vi "Obtain cycle time.vi"(8 "error in (no error)":errorcluster, 11 "Functional Imging UI Refs":T1) -> (0 "error out":errorcluster, 1 "Funct Acq Cycle time (sec)":dbl, 2 "Funct Acq cycle length (us)":dbl, 3 "Single funct.acq cycle time-stamps (us) [MovCor only]":dbl[](array[numeric]), 5 "MovCor enabled (value from header file)":bool)   [LabVIEW 2017]
uses:
  Typedefs/Functional Imging UI Refs.ctl
  xcontrol/XGrapher.xctl
  Typedefs/ROI selector array-ROI vis.ctl
  xcontrol/Interface VIs/Interface typedefs/Interface-ROI selection cluster.ctl
  Typedefs/ROI ID Enum.ctl
  Typedefs/Groups array referecne.ctl
  Typedefs/ROI visibility mode.ctl
panel:
  # "[Groups] is a Typedef"
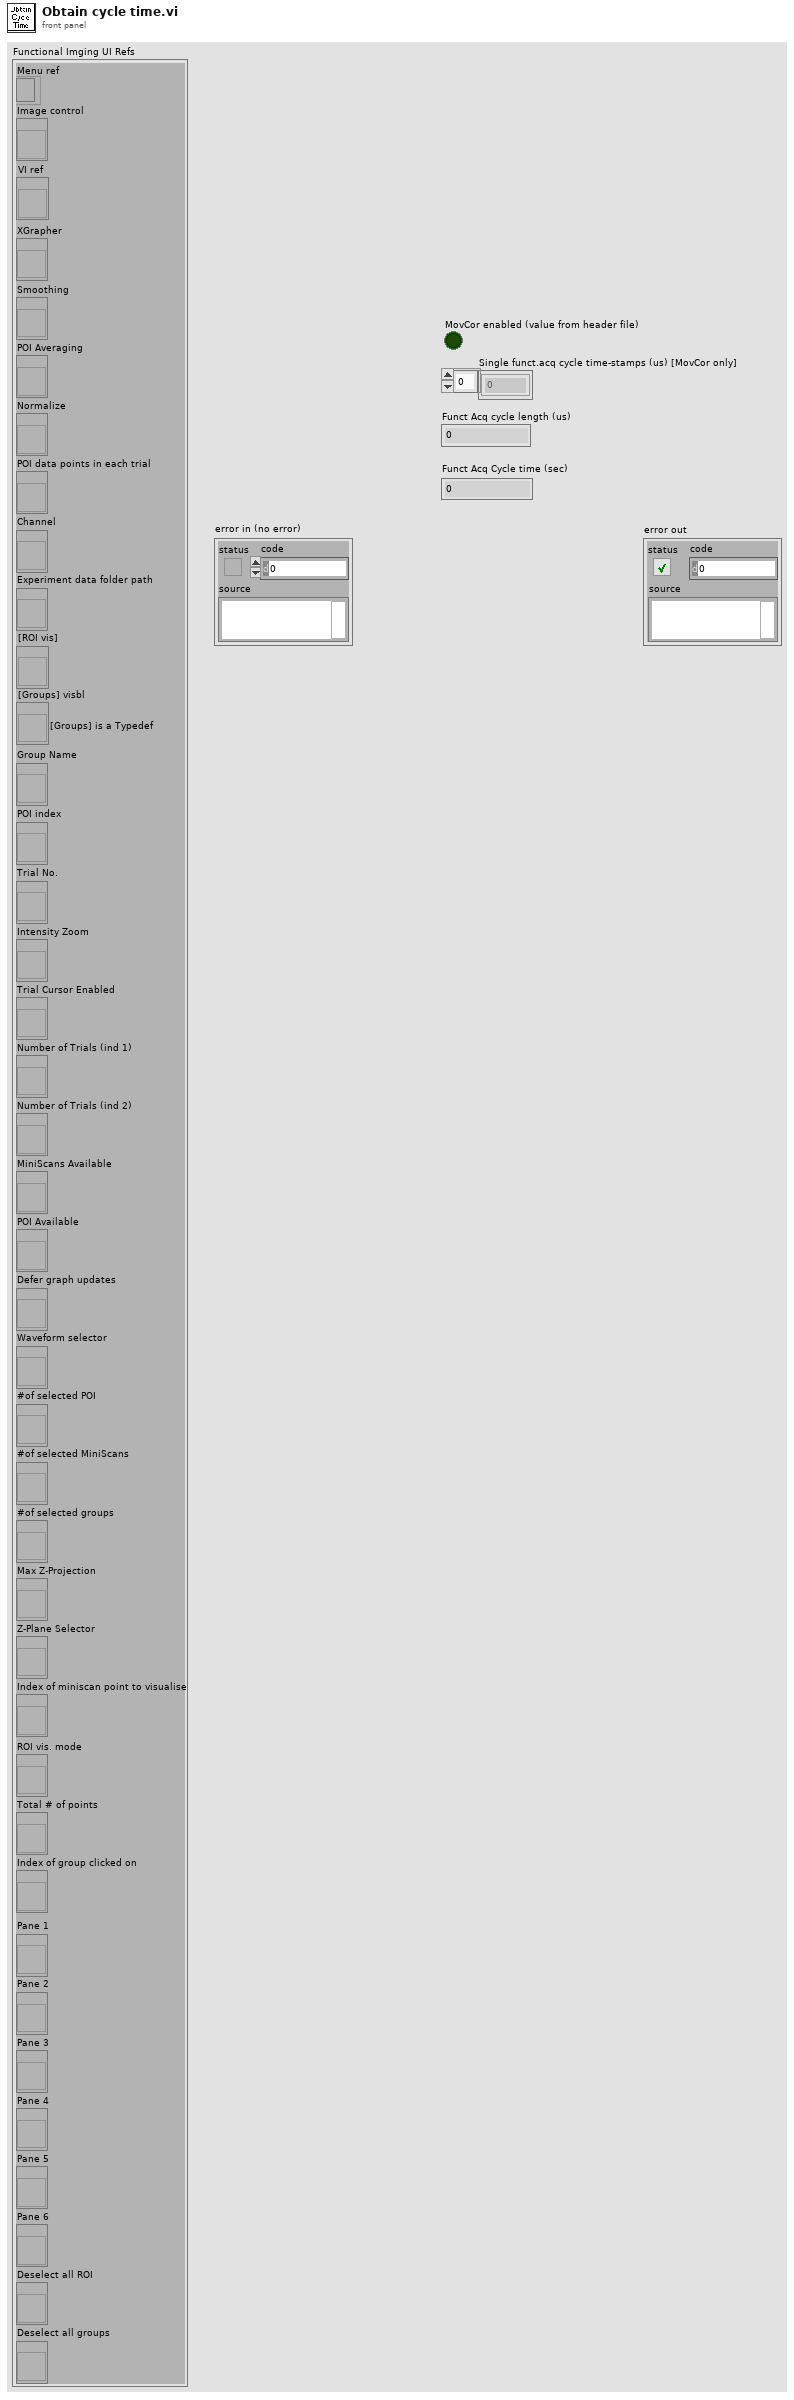
[diagram p1: front panel]
types:
  T1 = typedef "Functional Imging UI Refs.ctl" = cluster{"Menu ref":refnum<k9>, "Image control":refnum<vi>, "VI ref":refnum<vi>, "XGrapher":refnum<vi>, "Smoothing":refnum<vi>, "POI Averaging":refnum<vi>, "Normalize":refnum<vi>, "POI data points in each trial":refnum<vi>, "Channel":refnum<vi>, "Experiment data folder path":refnum<vi>, "[ROI vis]":refnum<vi>, "[Groups] visbl":T2, "Group Name":refnum<vi>, "POI index":refnum<vi>, "Trial No.":refnum<vi>, "Intensity Zoom":refnum<vi>, "Trial Cursor Enabled":refnum<vi>, "Number of Trials (ind 1)":refnum<vi>, "Number of Trials (ind 2)":refnum<vi>, "MiniScans Available":refnum<vi>, "POI Available":refnum<vi>, "Defer graph updates":refnum<vi>, "Waveform selector":refnum<vi>, "#of selected POI":refnum<vi>, "#of selected MiniScans":refnum<vi>, "#of selected groups":refnum<vi>, "Max Z-Projection":refnum<vi>, "Z-Plane Selector":refnum<vi>, "Index of miniscan point to visualise":refnum<vi>, "ROI vis. mode":refnum<vi>, "Total # of points":refnum<vi>, "Index of group clicked on":refnum<vi>, "Pane 1":refnum<vi>, "Pane 2":refnum<vi>, "Pane 3":refnum<vi>, "Pane 4":refnum<vi>, "Pane 5":refnum<vi>, "Pane 6":refnum<vi>, "Deselect all ROI":refnum<vi>, "Deselect all groups":refnum<vi>}
  T2 = typedef "Groups array referecne.ctl" = refnum<vi>
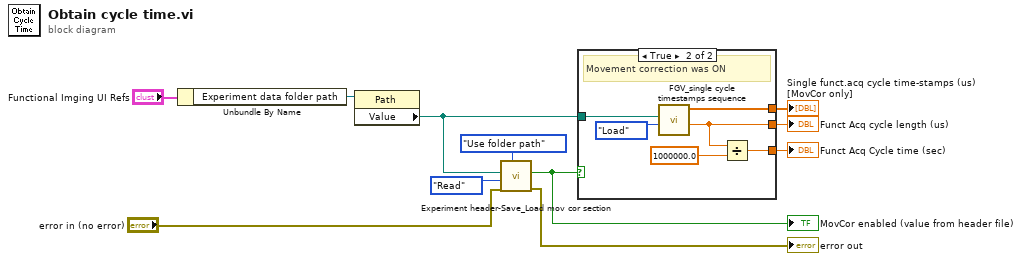
[diagram p0: block diagram]
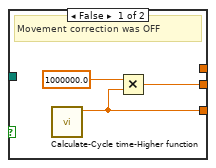
[diagram p2: hidden frame]
diagram:
  n1 = Unbundle By Name("Functional Imging UI Refs") -> ("Experiment data folder path"=w8:refnum<vi>)
  n2 = property on="Property Node" class="Path"(reference=w8) -> ("Value"=w6:path)  [unwired: 1 in, 2 out]
  n3 = call "Experiment header-Save_Load mov cor section.vi"("Input Mode (ref)"=enum16{"Use reference", "Use folder path"}."Use folder path", "error in (no error)"="error in (no error)", "Function"=enum16{"Write", "Read"}."Read", "Experiment folder path"=w6) -> ("error out"=→"error out":errorcluster, "MovCor enabled (value from header file)"=w3:bool)  [unwired: 5 in, 1 out]
  "MovCor enabled (value from header file)" <- w3
  n4 = case shown="True" w3 {
    tunnel: [w14 w17] -> w11
    tunnel: w6 -> [_ w19]
    tunnel: [_ w16] -> w5
    tunnel: [w13 w15] -> w4
    frame False {
      # "Movement correction was OFF"
      n5 = call "Calculate-Cycle time-Higher function.vi"() -> ("Cycle Time (s)"=w14:dbl)  [unwired: 11 in]
      n6 = Multiply(x=1000000.0, y=w14) -> (x*y=w13:dbl)
    }
    frame True {
      # "Movement correction was ON"
      n7 = call "FGV_single cycle timestamps sequence.vi"("Function"=enum16{"Read", "Write", "Load", "Save"}."Load", "Experiment folder path"=w19) -> ("Funct Acq cycle length (us)"=w15:dbl, "Single funct.acq cycle time-stamps (us)"=w16:dbl[])  [unwired: 8 in]
      n8 = Divide(x=w15, y=1000000.0) -> (x/y=w17:dbl)
    }
  }
  "Funct Acq Cycle time (sec)" <- w11
  "Single funct.acq cycle time-stamps (us) [MovCor only]" <- w5
  "Funct Acq cycle length (us)" <- w4
